vi "test Multi FPGA APU.vi"(8 "error in (no error)":errorcluster, 11 "TestCase in":refnum<class "Engine Simulation FPGA System Tests.lvclass">) -> (0 "error out":errorcluster, 3 "TestCase out":refnum<class "Engine Simulation FPGA System Tests.lvclass">)   [LabVIEW 2015, in "Engine Simulation FPGA System Tests.lvclass"]
uses:
  Engine Simulation FPGA System Tests.lvclass
  <vilib>/Utility/config.llb/Read Key (String).vi
  <vilib>/FPGAPlugInAG/PXIe-7822R/niLvFpga_Open_PXIe-7822R.vi
  <vilib>/rvi/interface/common/dynamic/niFpgaDynamicAddResources.vi
  <vilib>/Utility/error.llb/Error Cluster From Error Code.vi
  <vilib>/rvi/errors/niLvFpgaAdjustHostInterfaceError.vi
  <vilib>/FPGAPlugInAG/Dynamic/niLvFpga_Close_Dynamic.vi
  <vilib>/rvi/interface/nirviOpenFPGA/nirviOpenFPGA.xnode
  Assets/MultiFPGAAPUTest_PXIe-7822R.lvbitx
  <vilib>/rvi/interface/nirviReadWriteControl/nirviReadWriteControl.xnode
  <vilib>/rvi/interface/nirviCloseFPGA/nirviCloseFPGA.xnode
  <vilib>/addons/_JKI Toolkits/VI Tester/TestCase.llb/TestCase.lvclass
  NiFpgaLv.dll
  <vilib>/rvi/interface/Simulation/niFpgaSimulationCallBeginRW.vi
  <vilib>/Utility/config.llb/NI_LVConfig.lvlib
panel:
  in  "wait (ms)":u32
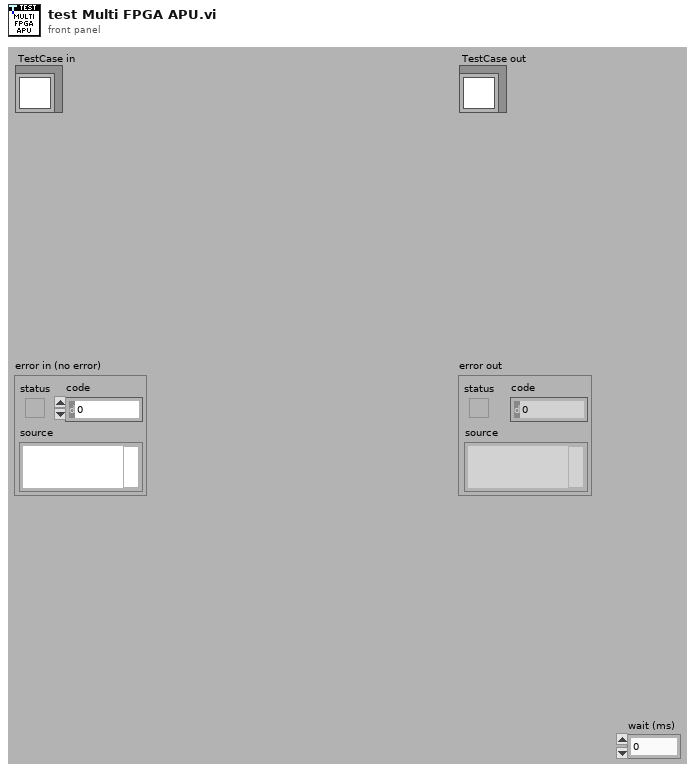
[diagram p1: front panel]
types:
  T1 = cluster{"desired speed":fxp<+/-,23,2>, "reset":bool}
  T2 = typedef "NI_LVConfig.lvlib/Config Data RefNum.ctl" = refnum<k1>
  T3 = cluster{"crank":u16, "cycle":u16, "actual speed":fxp<+/-,23,2>}
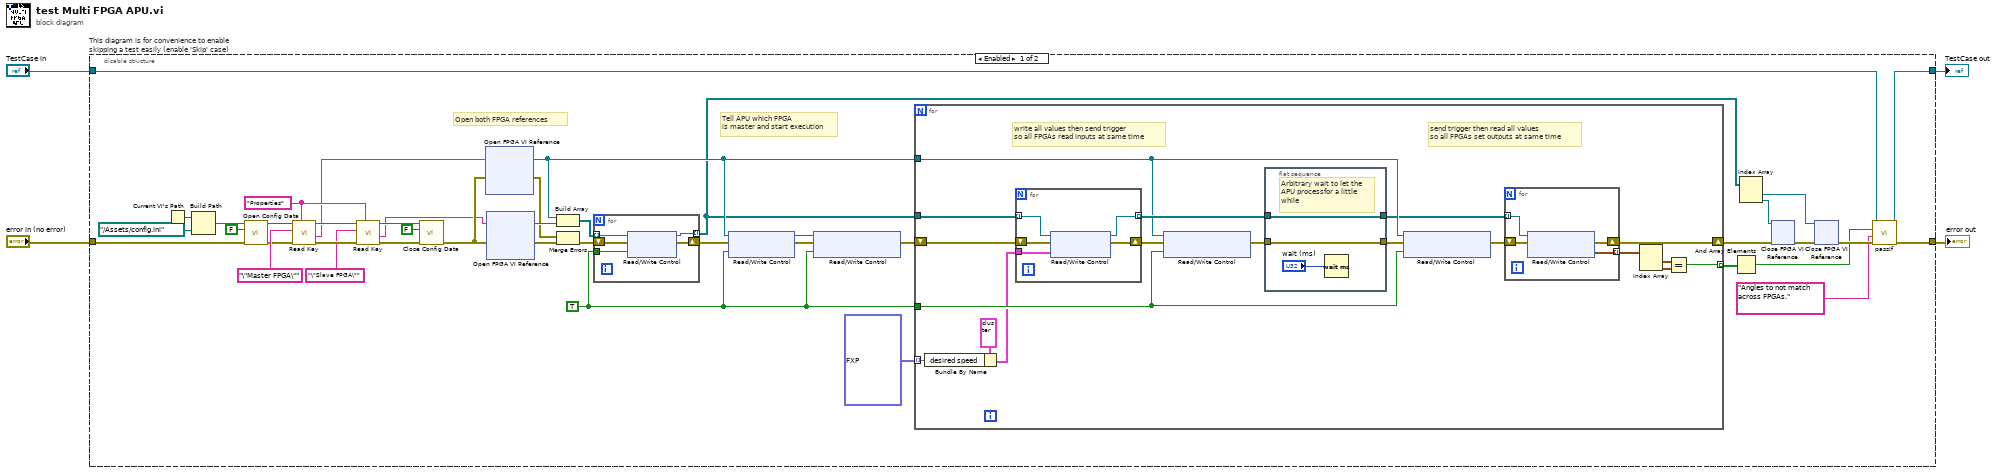
[diagram p0: block diagram]
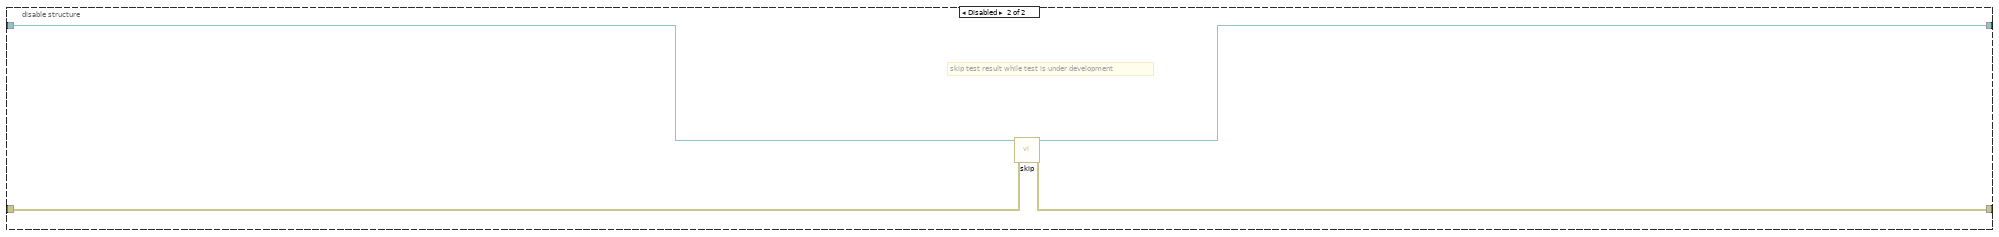
[diagram p2: hidden frame]
diagram:
  n1 = disable-structure "This diagram is for convenience to enable skipping a test easily (enable 'Skip' case)" shown="Enabled" {
    disable-tunnel: "TestCase in" -> [w27 w85]
    disable-tunnel: [w26 w83] -> w1
    disable-tunnel: [w24 w84] -> w3
    disable-tunnel: "error in (no error)" -> [w9 w82]
    frame Enabled {
      w17 = "Properties" ("section")
      w36 = TRUE ("master.apu 1")
      # "Tell APU which FPGA\nis master and start execution"
      # "Open both FPGA references"
      n2 = Current VI's Path() -> (path=w10:path)
      n3 = Build Path(base path=w10, name or relative path=path "../Assets/config.ini") -> (appended path=w12:path)
      n4 = call <vilib>:"Open Config Data.vi"("error in (no error)"=w9, "create file if necessary (T)"=FALSE, "configuration file path"=w12) -> ("error out"=w15:errorcluster, "refnum"=w14:T2)  [unwired: 6 in, 1 out]
      n5 = call-poly <vilib>:"Read Key.vi"("section"=w17, "error in (no error)"=w15, "key"="\"Master FPGA\"", "refnum"=w14) -> ("error out"=w23:errorcluster, "value"=w7:string, "refnum out"=w18:T2)  [unwired: 4 in, 1 out]
      n6 = call-poly <vilib>:"Read Key.vi"("section"=w17, "error in (no error)"=w23, "key"="\"Slave FPGA\"", "refnum"=w18) -> ("error out"=w20:errorcluster, "value"=w6:string, "refnum out"=w21:T2)  [unwired: 4 in, 1 out]
      n7 = call <vilib>:"Close Config Data.vi"("error in (no error)"=w20, "write file if changed (T)"=FALSE, "refnum"=w21) -> ("error out"=w8:errorcluster)  [unwired: 7 in, 1 out]
      n8 = xnode "Open FPGA VI Reference"("error in"=w8, "resource name"=w7) -> ("FPGA VI Reference Out"=w37:refnum<k20>, "error out"=w45:errorcluster)
      n9 = xnode "Open FPGA VI Reference"("error in"=w8, "resource name"=w6) -> ("FPGA VI Reference Out"=w46:refnum<k20>, "error out"=w44:errorcluster)
      n10 = Build Array(w37, w46) -> (w42:refnum<k20>[])
      n11 = Merge Errors(w45, w44) -> (w43:errorcluster)
      n12 = for {
        tunnel: w42 -> [w81] mode=indexing
        tunnel: [w80] -> w33 mode=indexing
        shift-right: [w79] -> w41
        shift-left: w43 -> [w78]
        tunnel: w36 -> [w77]
        n13 = xnode "Read/Write Control"("FPGA VI Reference In"=w81, "error in"=w78, "go.apu 1"=w77) -> ("FPGA VI Reference Out"=w80:refnum<k20>, "error out"=w79:errorcluster)
      }
      n14 = xnode "Read/Write Control"("FPGA VI Reference In"=w37, "error in"=w41, "master.apu 1"=w36) -> ("FPGA VI Reference Out"=w39:refnum<k20>, "error out"=w40:errorcluster)
      n15 = xnode "Read/Write Control"("FPGA VI Reference In"=w39, "error in"=w40, "send trigger.apu 1"=w36) -> ("error out"=w38:errorcluster)  [unwired: 1 out]
      n16 = for {
        shift-right: [w52] -> w35
        shift-left: w38 -> [w64]
        tunnel: w33 -> [w63]
        tunnel: w37 -> [w58]
        tunnel: w36 -> [w57]
        tunnel: fxp<+/-,23,2>[] [0.0, 1.0, 1.1999998092651367, 1.9999995231628418, 1.5] -> [w50] mode=indexing
        tunnel: [w47] -> w29 mode=indexing
        # "send trigger then read all values\nso all FPGAs set outputs at same time"
        # "write all values then send trigger\nso all FPGAs read inputs at same time"
        n17 = Bundle By Name(cluster=T1 {"desired speed"=0.0, "reset"=FALSE} ("input.apu 1"), "desired speed"=w50) -> (w49:T1)
        n18 = for {
          shift-right: [w76] -> w62
          shift-left: w64 -> [w75]
          tunnel: w63 -> [w74] mode=indexing
          tunnel: [w73] -> w60 mode=indexing
          tunnel: w49 -> [w72]
          n19 = xnode "Read/Write Control"("FPGA VI Reference In"=w74, "error in"=w75, "input.apu 1"=w72) -> ("FPGA VI Reference Out"=w73:refnum<k20>, "error out"=w76:errorcluster)
        }
        n20 = xnode "Read/Write Control"("FPGA VI Reference In"=w58, "error in"=w62, "send trigger.apu 1"=w57) -> ("error out"=w61:errorcluster)  [unwired: 1 out]
        n21 = flat-sequence {
          tunnel: w61 -> [w70]
          tunnel: [w70] -> w59
          tunnel: w60 -> [w69]
          tunnel: [w69] -> w55
          frame #0 {
            # "Arbitrary wait to let the\nAPU processfor a little\nwhile"
            n22 = Wait (ms)(milliseconds to wait="wait (ms)") -> ()  [unwired: 1 out]
          }
        }
        n23 = xnode "Read/Write Control"("FPGA VI Reference In"=w58, "error in"=w59, "send trigger.apu 1"=w57) -> ("error out"=w56:errorcluster)  [unwired: 1 out]
        n24 = for {
          shift-right: [w67] -> w52
          shift-left: w56 -> [w68]
          tunnel: [w66] -> w48 mode=indexing
          tunnel: w55 -> [w65] mode=indexing
          n25 = xnode "Read/Write Control"("FPGA VI Reference In"=w65, "error in"=w68) -> ("error out"=w67:errorcluster, "output.apu 1"=w66:T3)  [unwired: 1 out]
        }
        n26 = Index Array(array=w48) -> (element #1=w54:T3, element #2=w53:T3)  [unwired: 2 in]
        n27 = Equal?(x=w54, y=w53) -> (x = y?=w47:bool)
      }
      n28 = And Array Elements(Boolean array=w29) -> (logical AND=w25:bool)
      n29 = Index Array(array=w33) -> (element #1=w31:refnum<k20>, element #2=w32:refnum<k20>)  [unwired: 2 in]
      n30 = xnode "Close FPGA VI Reference"("FPGA VI Reference In"=w32, "error in"=w35) -> ("error out"=w34:errorcluster)
      n31 = xnode "Close FPGA VI Reference"("FPGA VI Reference In"=w31, "error in"=w34) -> ("error out"=w28:errorcluster)
      n32 = call-dynamic "passIf.vi"("error in (no error)"=w28, "message (\"\")"="Angles to not match across FPGAs." ("message (\"\")"), "pass"=w25, "TestCase in"=w27) -> ("error out"=w24:errorcluster, "TestCase out"=w26:refnum<class "Engine Simulation FPGA System Tests.lvclass">)  [unwired: 6 in]
    }
    frame Disabled {
      # "skip test result while test is under development"
      n33 = call <vilib>:"skip.vi"("error in (no error)"=w82, "TestCase in"=w85) -> ("error out"=w84:errorcluster, "TestCase out"=w83:refnum<class "Engine Simulation FPGA System Tests.lvclass">)  [unwired: 8 in]
    }
  }
  "error out" <- w3
  "TestCase out" <- w1
